vi "RT Main - Multi Thread.vi"() -> ()   [LabVIEW 2024]
uses:
  Driver/Source/Typedefs/GE 5565PIORC.Typedef.DMA Transfer Spec.ctl
  Driver/Source/Typedefs/GE 5565PIORC.Typedef.DMA Block Descriptor.ctl
  Driver/Source/Typedefs/GE 5565PIORC.Typedef.DMA Block Descriptor Params.ctl
  Driver/Source/Typedefs/GE 5565PIORC.Typedef.DMA Wait Mode.ctl
  <vilib>/Utility/RT CPU Load.ctl
  <vilib>/Platform/TimedLoop/XDataNode/timing_clust.ctl
  <vilib>/Platform/TimedLoop/XDataNode/nitl_modes.ctl
  <vilib>/Platform/TimedLoop/XDataNode/wakeup.ctl
  Driver/Source/GE 5565PIORC.lvclass/GE 5565PIORC.ctl
  Driver/Source/Methods/GE 5565PIORC.DMA.Create Transfer (Block).vi
  Driver/Source/Methods/GE 5565PIORC.DMA.Get Transfer Components (Block).vi
  Driver/Source/Methods/GE 5565PIORC.DMA.Block.Write (DBL).vi
  Driver/Source/Methods/GE 5565PIORC.DMA.Block.Read (DBL).vi
  Driver/Source/Properties/Registers/GE 5565PIORC.Registers.LAS1RR.PCI Address Range.Get.vi
  Driver/Source/Methods/GE 5565PIORC.PXI Interrupts.Enable.vi
  Driver/Source/Properties/Registers/GE 5565PIORC.Registers.DMACSR0.Channel 0 Enable.Set.vi
  Driver/Source/Properties/Registers/GE 5565PIORC.Registers.INTCSR.Local DMA Channel 0 Interrupt Enable.Set.vi
  Driver/Source/Methods/GE 5565PIORC.DMA.Create Transfer (Scatter-Gather).vi
  Driver/Source/Properties/GE 5565PIORC.Read VISA MEMACC.vi
  <vilib>/Utility/error.llb/Clear Errors.vi
  Driver/Source/Properties/Registers/GE 5565PIORC.Registers.DMADPR0.Direction of Transfer.Set.vi
  Driver/Source/Properties/Registers/GE 5565PIORC.Registers.DMASIZ0.DMA Transfer Size.Set.vi
  Driver/Source/Methods/GE 5565PIORC.DMA.Size.vi
  Driver/Source/Properties/Registers/GE 5565PIORC.Registers.DMALADR0.Local Address Register.Set.vi
  Driver/Source/Properties/Registers/GE 5565PIORC.Registers.DMAMODE0.Scatter-Gather Mode.Set.vi
  Driver/Source/Properties/Registers/GE 5565PIORC.Registers.DMAPADR0.PCI Address Register.Set.vi
  Driver/Source/Methods/GE 5565PIORC.DMA.Scatter-Gather.Link Block Descriptors.vi
  Driver/Source/Methods/GE 5565PIORC.DMA.Scatter-Gather.Commit Linked Block Descriptors.vi
  Driver/Source/Properties/Registers/GE 5565PIORC.Registers.DMADPR0.Channel 0 First Descriptor Address.Set.vi
  Driver/Source/Methods/GE 5565PIORC.DMA.Get Transfer Components (Scatter-Gather).vi
  Driver/Source/Properties/Registers/GE 5565PIORC.Registers.DMACSR0.Channel 0 Start.Set.vi
  Driver/Source/Properties/Registers/GE 5565PIORC.Registers.DMACSR0.Channel 0 Clear Interrupt.Set.vi
  Driver/Source/Methods/GE 5565PIORC.DMA.Poll for Done Signal.vi
  Driver/Source/Methods/GE 5565PIORC.PXI Interrupts.Wait for Event.vi
  Driver/Source/Properties/Registers/GE 5565PIORC.Registers.Local Configuration.Read.vi
  Driver/Source/Properties/Registers/GE 5565PIORC.Registers.Local Configuration.Read (U32).vi
  Driver/Source/Properties/Registers/GE 5565PIORC.Registers.Local Configuration.Read (U8).vi
  Driver/Source/Properties/Registers/GE 5565PIORC.Registers.Local Configuration.Write.vi
  Driver/Source/Properties/Registers/GE 5565PIORC.Registers.Local Configuration.Write (U8).vi
  Driver/Source/Methods/GE 5565PIORC.Bit Manipulation.Set Bit.vi
  Driver/Source/Methods/GE 5565PIORC.Bit Manipulation.Set Bit (U8).vi
  Driver/Source/Properties/Registers/GE 5565PIORC.Registers.Local Configuration.Write (U32).vi
  Driver/Source/Methods/GE 5565PIORC.Bit Manipulation.Set Bit (U32).vi
  Driver/Source/Methods/GE 5565PIORC.DMA.Scatter-Gather.Set Descriptor Params.vi
  Driver/Source/Methods/GE 5565PIORC.DMA.Is Done.vi
  Driver/Source/Methods/GE 5565PIORC.Registers.Read.vi
  Driver/Source/Methods/GE 5565PIORC.Registers.Read (U32).vi
  Driver/Source/Methods/GE 5565PIORC.Registers.Read (U8).vi
  Driver/Source/Methods/GE 5565PIORC.Registers.Write.vi
  Driver/Source/Methods/GE 5565PIORC.Registers.Write (U8).vi
  Driver/Source/Methods/GE 5565PIORC.Registers.Write (U32).vi
  Driver/Source/Properties/Registers/GE 5565PIORC.Registers.DMACSR0.Channel 0 Inactive.Get.vi
  Driver/Source/Methods/GE 5565PIORC.Bit Manipulation.Get Bit.vi
  Driver/Source/Methods/GE 5565PIORC.Bit Manipulation.Get Bit (U8).vi
  Driver/Source/Methods/GE 5565PIORC.Round Up to Nearest 8.vi
  Driver/Source/Methods/GE 5565PIORC.Round Up to Nearest 16.vi
  Driver/Source/GE 5565PIORC.lvclass
  <vilib>/platform/TimedLoop/XDataNode/XDataNode.xnode
  <vilib>/Platform/TimedLoop/XDataNode/XDNodeRunTimeDep.lvlib
  <vilib>/NI_Real-Time Target Support.lvlib
panel:
  out "Write Delta T (ms)":u32
  out "Write Iteration":i32
  out "Prev Read Data":dbl[](array[numeric])
  in  "Read Count (DBLs)":u32
  in  "Write Count (DBLs)":u32
  in  "Reverse Data":bool
  in  "Stop if Different?":bool=TRUE
  out "data out size":i32
  out "Read Size":i32
  out "CPU loads":T1[](array[typedef]) {"ISR (%)" format="%#.2f"; "Idle (%)" format="%#.2f"; "Background (%)" format="%#.2f"; "Normal (%)" format="%#.2f"; "Above Normal (%)" format="%#.2f"; "High (%)" format="%#.2g"; "Timed Structures (%)" format="%#.2g"; "Time Critical (%)" format="%#.2g"; "Total (%)" format="%#.2g"}
  out "Diff Count":i32
  out "Read Delta T (ms)":u32
  out "Write Timeout":i16(graph)
  out "Read Timeout":i16(graph)
  in  "Write Offset (DBLs)":u32
  in  "Read Offset (DBLs)":u32
  out "Read Data":dbl[][](graph)
  in  "VISA resource name":refnum<visa-resource-name>="PXI17::11::INSTR"
  out "Read Iteration":i32
  in  "stop":bool
  out "Read Data":dbl[](array[numeric])
  in  "Write Data":dbl[](array[numeric])
  out "Write - DMA Transfer Spec":T2 {"Block Descriptors"."descriptor params"."data ptr (lower)" format="%.0x"; "Block Descriptors"."descriptor params"."data ptr (upper)" format="%.0x"; "Block Descriptors"."descriptor params"."data size" format="%.0x"; "Block Descriptors"."descriptor params"."next descriptor ptr" format="%.0x"; "Block Descriptors"."descriptor size" format="%08x"; "Block Descriptors"."descriptor ptr (RFM)" format="%08x"; "Block Descriptors"."descriptor ptr (VISA)" format="%08x"; "RFM offset" format="%08x"}
  out "Write Time Out?":bool
  out "error out":errorcluster
  out "Read Time Out?":bool
  in  "wait mode (polling)":T5
  out "Read - DMA Transfer Spec":T2 {"Block Descriptors"."descriptor params"."data ptr (lower)" format="%.0x"; "Block Descriptors"."descriptor params"."data ptr (upper)" format="%.0x"; "Block Descriptors"."descriptor params"."data size" format="%.0x"; "Block Descriptors"."descriptor params"."next descriptor ptr" format="%.0x"; "Block Descriptors"."descriptor size" format="%08x"; "Block Descriptors"."descriptor ptr (RFM)" format="%08x"; "Block Descriptors"."descriptor ptr (VISA)" format="%08x"; "RFM offset" format="%08x"}
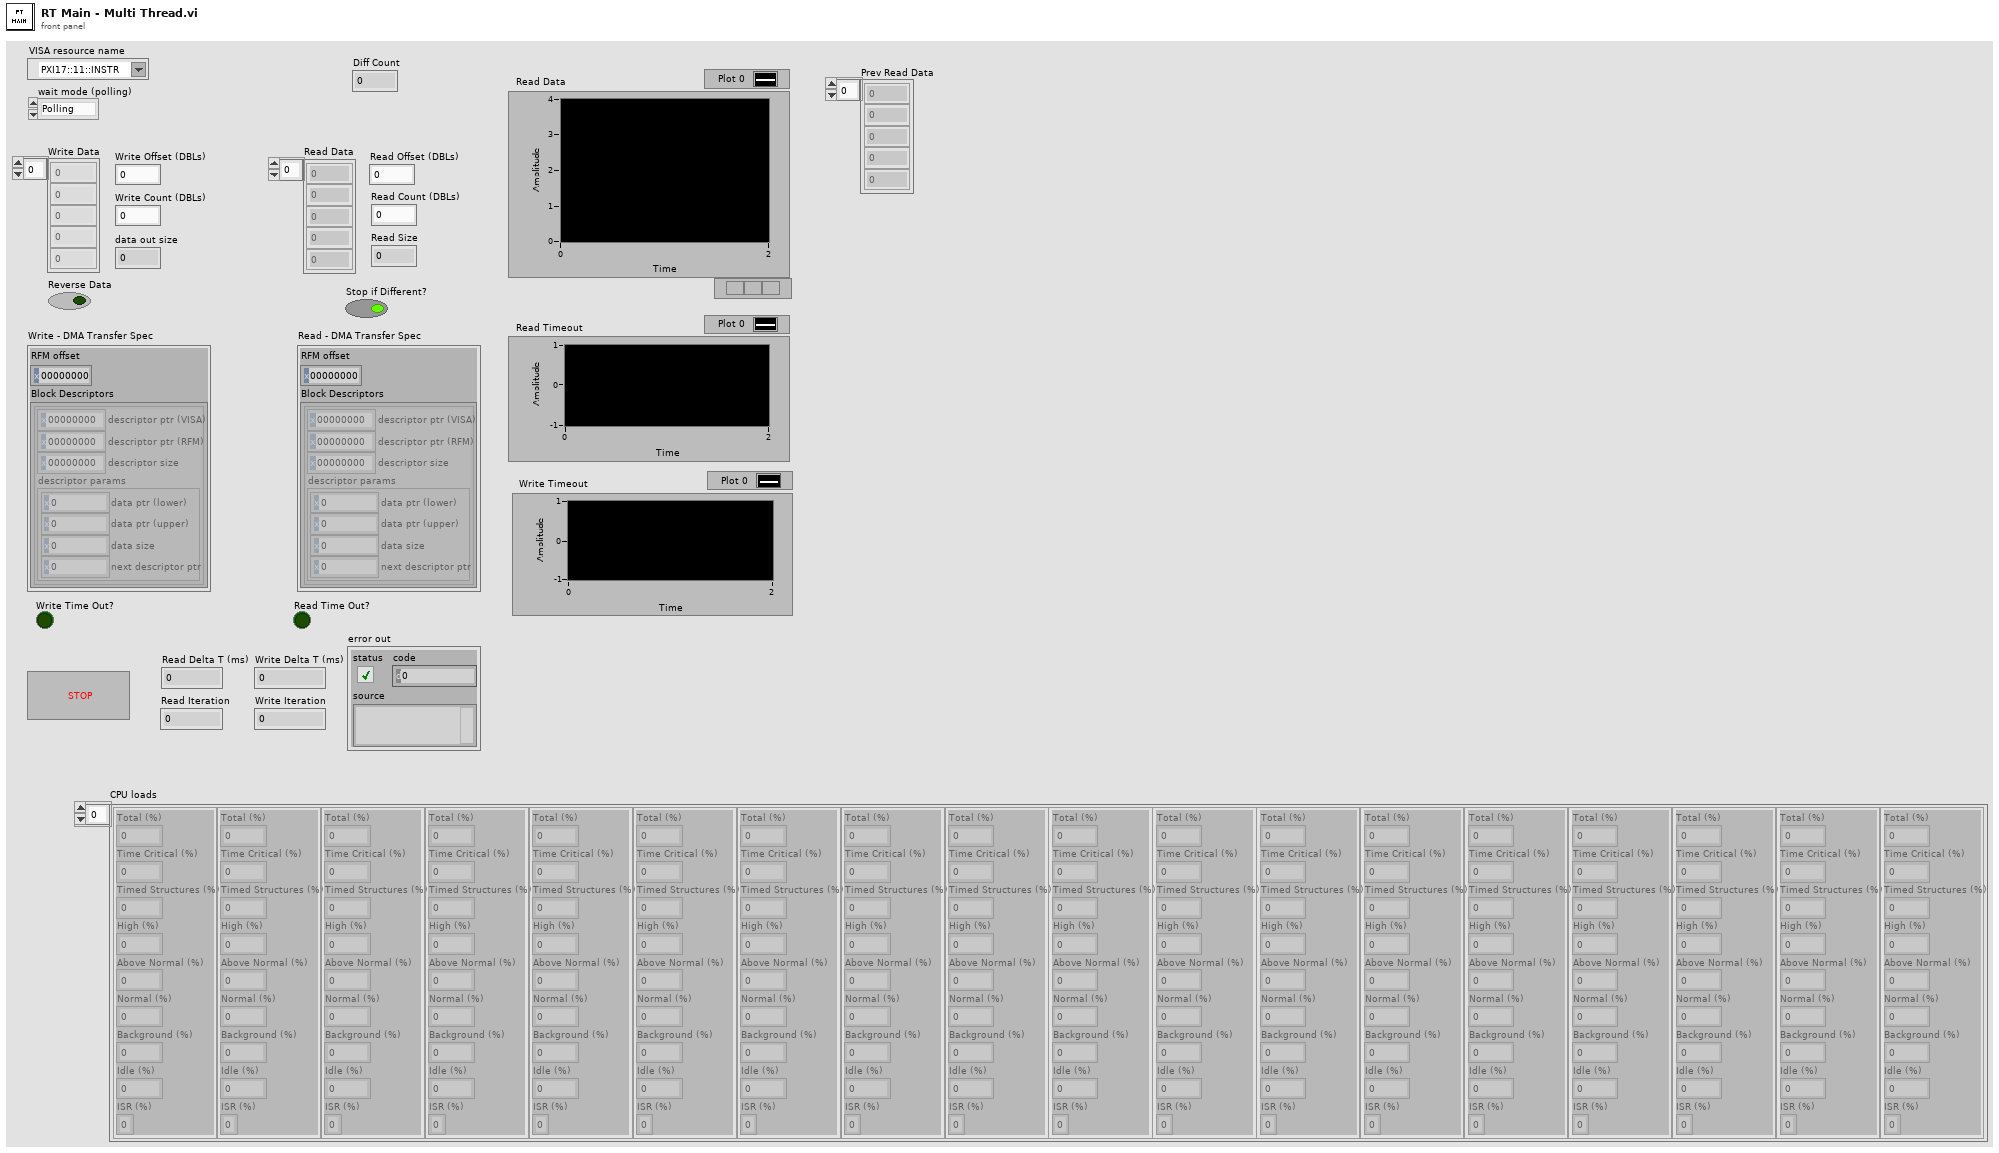
[diagram p1: front panel]
types:
  T1 = typedef "NI_Real-Time Target Support.lvlib/RT CPU Load.ctl" = cluster{"Total (%)":dbl, "Time Critical (%)":dbl, "Timed Structures (%)":dbl, "High (%)":dbl, "Above Normal (%)":dbl, "Normal (%)":dbl, "Background (%)":dbl, "Idle (%)":dbl, "ISR (%)":dbl}
  T2 = typedef "GE 5565PIORC.lvclass/GE 5565PIORC.Typedef.DMA Transfer Spec.ctl" = cluster{"RFM offset":u32, "Block Descriptors":T3[]}
  T3 = typedef "GE 5565PIORC.lvclass/GE 5565PIORC.Typedef.DMA Block Descriptor.ctl" = cluster{"descriptor ptr (VISA)":u32, "descriptor ptr (RFM)":u32, "descriptor size":u32, "descriptor params":T4}
  T4 = typedef "GE 5565PIORC.lvclass/GE 5565PIORC.Typedef.DMA Block Descriptor Params.ctl" = cluster{"data ptr (lower)":u32, "data ptr (upper)":u32, "data size":u32, "next descriptor ptr":u32}
  T5 = typedef "GE 5565PIORC.lvclass/GE 5565PIORC.Typedef.DMA Wait Mode.ctl" = enum16{"Polling", "Interrupt"}
  T6 = typedef "XDNodeRunTimeDep.lvlib/timing_clust.ctl" = cluster{"Expected End [f-1]":u64, "Actual End [f-1]":u64, "Finished Late? [f-1]":bool, "Expected End [i-1]":u64, "Actual End [i-1]":u64, "Finished Late? [i-1]":bool, "Expected Start [i]":u64, "Actual Start [i]":u64, "Expected Start [f]":u64, "Actual Start [f]":u64, "Source Name":string, "Structure Name":string, "Period":i64, "Deadline":i64, "Offset":i64, "Start":i64, "Priority":i32, "Timeout":i32, "Mode":T7, "Wakeup Reason":T8, "Error":errorcluster, "Source Type":string, "Secondary Source Type":string, "Global End Time":u64, "Global Start Time":u64, "Frame Duration":u64, "Iteration Duration":u64, "Assigned CPU":i32, "I/O Scan Engine Mode":u32}
  T7 = typedef "XDNodeRunTimeDep.lvlib/nitl_modes.ctl" = enum32{"No Change", "Process missed periods, maintain original phase", "Discard missed periods, maintain original phase", "Process missed periods, ignore original phase", "Discard missed periods, ignore original phase"}
  T8 = typedef "XDNodeRunTimeDep.lvlib/wakeup.ctl" = enum32{"Normal", "Aborted", "Asynchronous wakeup", "Timing source error", "Timed loop error", "Timeout"}
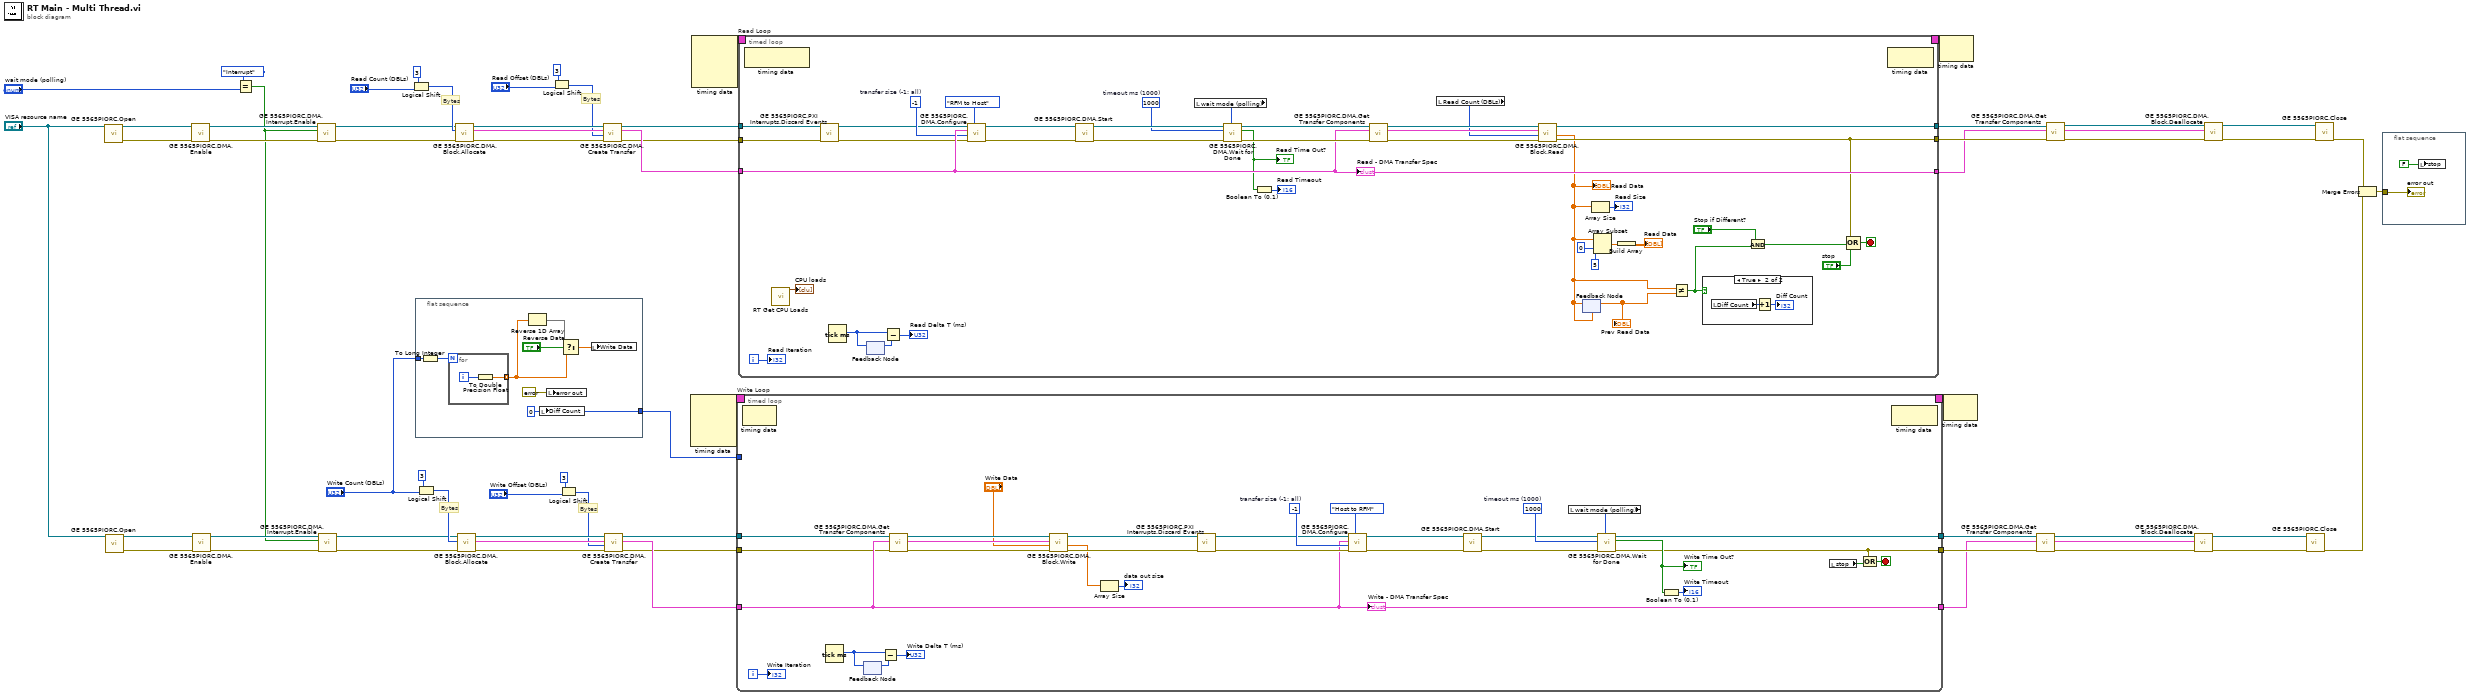
[diagram p0: block diagram]
diagram:
  # "Bytes"
  # "Bytes"
  # "Bytes"
  # "Bytes"
  n1 = call "GE 5565PIORC.Open.vi"("VISA resource name"="VISA resource name") -> ("error out"=w63:errorcluster, "GE 5565PIORC"=w64:refnum<class "GE 5565PIORC.lvclass">)  [unwired: 9 in]
  n2 = call "GE 5565PIORC.Open.vi"("VISA resource name"="VISA resource name") -> ("error out"=w7:errorcluster, "GE 5565PIORC"=w8:refnum<class "GE 5565PIORC.lvclass">)  [unwired: 9 in]
  n3 = call "GE 5565PIORC.DMA.Enable.vi"("error in (no error)"=w63, "GE 5565PIORC in"=w64) -> ("error out"=w59:errorcluster, "GE 5565PIORC out"=w60:refnum<class "GE 5565PIORC.lvclass">)  [unwired: 8 in]
  n4 = call "GE 5565PIORC.DMA.Enable.vi"("error in (no error)"=w7, "GE 5565PIORC in"=w8) -> ("error out"=w5:errorcluster, "GE 5565PIORC out"=w6:refnum<class "GE 5565PIORC.lvclass">)  [unwired: 8 in]
  n5 = Equal?(x=GE_5565PIORC.Typedef.DMA_Wait_Mode."Interrupt" ("wait mode (polling)"), y="wait mode (polling)") -> (x = y?=w2:bool)
  n6 = call "GE 5565PIORC.DMA.Interrupt.Enable.vi"("error in (no error)"=w59, "enable (T)"=w2, "GE 5565PIORC in"=w60) -> ("error out"=w9:errorcluster, "GE 5565PIORC out"=w10:refnum<class "GE 5565PIORC.lvclass">)  [unwired: 7 in]
  n7 = call "GE 5565PIORC.DMA.Interrupt.Enable.vi"("error in (no error)"=w5, "enable (T)"=w2, "GE 5565PIORC in"=w6) -> ("error out"=w3:errorcluster, "GE 5565PIORC out"=w4:refnum<class "GE 5565PIORC.lvclass">)  [unwired: 7 in]
  n8 = Logical Shift(y=i16 3, x="Read Count (DBLs)") -> (x << y=w47:u32)
  n9 = flat-sequence {
    tunnel: [w72] -> w32
    tunnel: "Write Count (DBLs)" -> [w66]
    frame #0 {
      w72 = 0 ("Diff Count")
      n10 = To Long Integer(number=w66) -> (32bit integer=w67:i32)
      n11 = for {
        N: w67 -> [_]
        tunnel: [w73] -> w70 mode=indexing
        i -> [w74]
        n12 = To Double Precision Float(number=w74) -> (double precision float=w73:dbl)
      }
      n13 = Reverse 1D Array(array=w70) -> (reversed array=w71:dbl[])
      n14 = local write "Diff Count"(w72) -> ()
      n15 = local write "error out"(errorcluster {"status"=FALSE, "code"=0, "source"=""} ("error out")) -> ()
      n16 = Select(t=w71, s="Reverse Data", f=w70) -> (s? t:f=w68:dbl[])
      n17 = local write "Write Data"(w68) -> ()
    }
  }
  n18 = Logical Shift(y=i16 3, x="Write Count (DBLs)") -> (x << y=w44:u32)
  n19 = call "GE 5565PIORC.DMA.Block.Allocate.vi"("error in (no error)"=w9, "size in bytes"=w47, "GE 5565PIORC in"=w10) -> ("error out"=w62:errorcluster, "Block Descriptor"=w61:T3, "GE 5565PIORC out"=w55:refnum<class "GE 5565PIORC.lvclass">)  [unwired: 6 in]
  n20 = call "GE 5565PIORC.DMA.Block.Allocate.vi"("error in (no error)"=w3, "size in bytes"=w44, "GE 5565PIORC in"=w4) -> ("error out"=w51:errorcluster, "Block Descriptor"=w50:T3, "GE 5565PIORC out"=w52:refnum<class "GE 5565PIORC.lvclass">)  [unwired: 6 in]
  n21 = Logical Shift(y=i16 3, x="Read Offset (DBLs)") -> (x << y=w41:u32)
  n22 = Logical Shift(y=i16 3, x="Write Offset (DBLs)") -> (x << y=w38:u32)
  n23 = call-poly "GE 5565PIORC.DMA.Create Transfer.vi"("error in (no error)"=w62, "RFM offset"=w41, "Block Descriptor"=w61, "GE 5565PIORC in"=w55) -> ("error out"=w13:errorcluster, "DMA Transfer Spec"=w56:T2, "GE 5565PIORC out"=w14:refnum<class "GE 5565PIORC.lvclass">)  [unwired: 4 in, 1 out]
  n24 = call-poly "GE 5565PIORC.DMA.Create Transfer.vi"("error in (no error)"=w51, "RFM offset"=w38, "Block Descriptor"=w50, "GE 5565PIORC in"=w52) -> ("error out"=w11:errorcluster, "DMA Transfer Spec"=w33:T2, "GE 5565PIORC out"=w12:refnum<class "GE 5565PIORC.lvclass">)  [unwired: 4 in, 1 out]
  n25 = node-c288() -> (w35:T6)  [unwired: 4 in]
  n26 = node-c288() -> (w58:T6)  [unwired: 4 in]
  n27 = timed-loop "Write Loop" {
    timing: w35 -> [_]
    timing-out: [_] -> w34
    tunnel: w33 -> [w84]
    tunnel: [w85] -> w20
    tunnel: [w76] -> w19
    tunnel: [w84] -> w18
    tunnel: w32 -> [_]
    tunnel: w12 -> [w83]
    tunnel: w11 -> [w82]
    i -> [w81]
    stop <- w75 stop-if-true
    w96 = -1  # transfer size (-1: all)
    w103 = u32 1000  # timeout ms (1000)
    n28 = node-c288() -> ()  [unwired: 1 in, 1 out]
    n29 = Tick Count (ms)() -> (millisecond timer value=w80:u32)
    n30 = feedback #1() -> (w79:u32)  [unwired: 1 in]
    n31 = feedback-in #1(w80) -> ()
    n32 = Subtract(x=w80, y=w79) -> (x-y=→"Write Delta T (ms)":u32)
    n33 = call-poly "GE 5565PIORC.DMA.Get Transfer Components.vi"("error in (no error)"=w82, "DMA Transfer Spec in"=w84, "GE 5565PIORC in"=w83) -> ("error out"=w91:errorcluster, "Block Descriptor"=w97:T3, "GE 5565PIORC out"=w92:refnum<class "GE 5565PIORC.lvclass">)  [unwired: 5 in, 1 out]
    n34 = call-poly "GE 5565PIORC.DMA.Block.Write.vi"("error in (no error)"=w91, "data"="Write Data", "Block Descriptor in"=w97, "GE 5565PIORC in"=w92) -> ("error out"=w105:errorcluster, "data out"=w86:dbl[], "GE 5565PIORC out"=w104:refnum<class "GE 5565PIORC.lvclass">)  [unwired: 4 in, 1 out]
    n35 = Array Size(array=w86) -> (size(s)=→"data out size":i32)
    n36 = call "GE 5565PIORC.PXI Interrupts.Discard Events.vi"("error in (no error)"=w105, "GE 5565PIORC in"=w104) -> ("error out"=w93:errorcluster, "GE 5565PIORC out"=w94:refnum<class "GE 5565PIORC.lvclass">)  [unwired: 8 in]
    n37 = call "GE 5565PIORC.DMA.Configure.vi"("transfer direction"=enum16{"Host to RFM", "RFM to Host"}."Host to RFM", "error in (no error)"=w93, "transfer size (-1: all)"=w96, "DMA Transfer Spec"=w84, "GE 5565PIORC in"=w94) -> ("error out"=w98:errorcluster, "GE 5565PIORC out"=w100:refnum<class "GE 5565PIORC.lvclass">)  [unwired: 5 in]
    n38 = call "GE 5565PIORC.DMA.Start.vi"("error in (no error)"=w98, "GE 5565PIORC in"=w100) -> ("error out"=w99:errorcluster, "GE 5565PIORC out"=w101:refnum<class "GE 5565PIORC.lvclass">)  [unwired: 8 in]
    n39 = local read "wait mode (polling)"() -> (w102:T5)
    n40 = call "GE 5565PIORC.DMA.Wait for Done.vi"("wait mode (polling)"=w102, "error in (no error)"=w99, "timeout ms (1000)"=w103, "GE 5565PIORC in"=w101) -> ("error out"=w76:errorcluster, "timed out?"=w88:bool, "GE 5565PIORC out"=w85:refnum<class "GE 5565PIORC.lvclass">)  [unwired: 5 in]
    "Write Time Out?" <- w88
    n41 = Boolean To (0,1)(Boolean=w88) -> (0, 1=→"Write Timeout":i16)
    n42 = local read "stop"() -> (w77:bool)
    n43 = Compound Arithmetic op=OR(w76, w77) -> (w75:bool)
    n44 = node-c288() -> ()  [unwired: 1 in, 1 out]
    "Write - DMA Transfer Spec" <- w84
    "Write Iteration" <- w81
  }
  n45 = timed-loop "Read Loop" {
    timing: w58 -> [_]
    timing-out: [_] -> w57
    tunnel: w14 -> [w115]
    tunnel: w13 -> [w114]
    tunnel: w56 -> [w140]
    tunnel: [w140] -> w26
    tunnel: [w113] -> w37
    tunnel: [w111] -> w36
    i -> [w137]
    stop <- w138 stop-if-true
    w123 = -1  # transfer size (-1: all)
    w139 = u32 1000  # timeout ms (1000)
    n46 = node-c288() -> ()  [unwired: 1 in, 1 out]
    n47 = call <vilib>:"RT Get CPU Loads.vi"() -> ("CPU loads"=→"CPU loads":T1[])  [unwired: 10 in, 1 out]
    n48 = call "GE 5565PIORC.PXI Interrupts.Discard Events.vi"("error in (no error)"=w114, "GE 5565PIORC in"=w115) -> ("error out"=w121:errorcluster, "GE 5565PIORC out"=w122:refnum<class "GE 5565PIORC.lvclass">)  [unwired: 8 in]
    n49 = Tick Count (ms)() -> (millisecond timer value=w130:u32)
    n50 = feedback #2() -> (w129:u32)  [unwired: 1 in]
    n51 = feedback-in #2(w130) -> ()
    n52 = Subtract(x=w130, y=w129) -> (x-y=→"Read Delta T (ms)":u32)
    n53 = call "GE 5565PIORC.DMA.Configure.vi"("transfer direction"=enum16{"Host to RFM", "RFM to Host"}."RFM to Host", "error in (no error)"=w121, "transfer size (-1: all)"=w123, "DMA Transfer Spec"=w140, "GE 5565PIORC in"=w122) -> ("error out"=w145:errorcluster, "GE 5565PIORC out"=w147:refnum<class "GE 5565PIORC.lvclass">)  [unwired: 5 in]
    n54 = call "GE 5565PIORC.DMA.Start.vi"("error in (no error)"=w145, "GE 5565PIORC in"=w147) -> ("error out"=w144:errorcluster, "GE 5565PIORC out"=w146:refnum<class "GE 5565PIORC.lvclass">)  [unwired: 8 in]
    n55 = local read "wait mode (polling)"() -> (w143:T5)
    n56 = call "GE 5565PIORC.DMA.Wait for Done.vi"("wait mode (polling)"=w143, "error in (no error)"=w144, "timeout ms (1000)"=w139, "GE 5565PIORC in"=w146) -> ("error out"=w141:errorcluster, "timed out?"=w132:bool, "GE 5565PIORC out"=w142:refnum<class "GE 5565PIORC.lvclass">)  [unwired: 5 in]
    "Read Time Out?" <- w132
    n57 = Boolean To (0,1)(Boolean=w132) -> (0, 1=→"Read Timeout":i16)
    n58 = call-poly "GE 5565PIORC.DMA.Get Transfer Components.vi"("error in (no error)"=w141, "DMA Transfer Spec in"=w140, "GE 5565PIORC in"=w142) -> ("error out"=w134:errorcluster, "Block Descriptor"=w133:T3, "GE 5565PIORC out"=w135:refnum<class "GE 5565PIORC.lvclass">)  [unwired: 5 in, 1 out]
    n59 = local read "Read Count (DBLs)"() -> (w116:u32)
    n60 = call-poly "GE 5565PIORC.DMA.Block.Read.vi"("error in (no error)"=w134, "count"=w116, "Block Descriptor in"=w133, "GE 5565PIORC in"=w135) -> ("error out"=w111:errorcluster, "data out"=w109:dbl[], "GE 5565PIORC out"=w113:refnum<class "GE 5565PIORC.lvclass">)  [unwired: 4 in, 1 out]
    "Read Data" <- w109
    n61 = feedback #3(w109) -> (w108:dbl[])
    "Prev Read Data" <- w108
    n62 = feedback-in #3(w109) -> ()
    n63 = Array Size(array=w109) -> (size(s)=→"Read Size":i32)
    n64 = Array Subset(array=w109, index=0, length=5) -> (w125:dbl[])
    n65 = Build Array(w125) -> (→"Read Data":dbl[][])
    n66 = Not Equal?(x=w109, y=w108) -> (x != y?=w117:bool)
    n67 = case shown="True" w117 {
      frame False {
      }
      frame True {
        n68 = local read "Diff Count"() -> (w151:i32)
        n69 = Increment(x=w151) -> (x+1=→"Diff Count":i32)
      }
    }
    n70 = And(x="Stop if Different?", y=w117) -> (x .and. y?=w112:bool)
    n71 = Compound Arithmetic op=OR(w111, w112, "stop") -> (w138:bool)
    n72 = node-c288() -> ()  [unwired: 1 in, 1 out]
    "Read - DMA Transfer Spec" <- w140
    "Read Iteration" <- w137
  }
  n73 = node-c288(w57) -> ()  [unwired: 1 out]
  n74 = node-c288(w34) -> ()  [unwired: 1 out]
  n75 = call-poly "GE 5565PIORC.DMA.Get Transfer Components.vi"("error in (no error)"=w19, "DMA Transfer Spec in"=w18, "GE 5565PIORC in"=w20) -> ("error out"=w23:errorcluster, "Block Descriptor"=w24:T3, "GE 5565PIORC out"=w25:refnum<class "GE 5565PIORC.lvclass">)  [unwired: 5 in, 1 out]
  n76 = call-poly "GE 5565PIORC.DMA.Get Transfer Components.vi"("error in (no error)"=w36, "DMA Transfer Spec in"=w26, "GE 5565PIORC in"=w37) -> ("error out"=w29:errorcluster, "Block Descriptor"=w30:T3, "GE 5565PIORC out"=w31:refnum<class "GE 5565PIORC.lvclass">)  [unwired: 5 in, 1 out]
  n77 = call "GE 5565PIORC.DMA.Block.Deallocate.vi"("error in (no error)"=w23, "Block Descriptor"=w24, "GE 5565PIORC in"=w25) -> ("error out"=w21:errorcluster, "GE 5565PIORC out"=w22:refnum<class "GE 5565PIORC.lvclass">)  [unwired: 7 in]
  n78 = call "GE 5565PIORC.DMA.Block.Deallocate.vi"("error in (no error)"=w29, "Block Descriptor"=w30, "GE 5565PIORC in"=w31) -> ("error out"=w27:errorcluster, "GE 5565PIORC out"=w28:refnum<class "GE 5565PIORC.lvclass">)  [unwired: 7 in]
  n79 = call "GE 5565PIORC.Close.vi"("error in (no error)"=w21, "GE 5565PIORC in"=w22) -> ("error out"=w16:errorcluster)  [unwired: 8 in, 1 out]
  n80 = call "GE 5565PIORC.Close.vi"("error in (no error)"=w27, "GE 5565PIORC in"=w28) -> ("error out"=w17:errorcluster)  [unwired: 8 in, 1 out]
  n81 = Merge Errors(w17, w16) -> (w15:errorcluster)
  n82 = flat-sequence {
    tunnel: w15 -> [w153]
    frame #0 {
      n83 = local write "stop"(FALSE) -> ()
      "error out" <- w153
    }
  }
